vi "FPGA_w8randLEDs.vi"() -> ()   [LabVIEW 2012]
uses:
  <vilib>/Platform/TimedLoop/XDataNode/timing_clust.ctl
  <vilib>/Platform/TimedLoop/XDataNode/nitl_modes.ctl
  <vilib>/Platform/TimedLoop/XDataNode/wakeup.ctl
  <vilib>/rvi/DataTransferAndStorage/Container/Common/niFpgaContainerMetaDataKey.ctl
  <vilib>/rvi/DataTransferAndStorage/Container/Common/niFpgaContainerState.ctl
  <vilib>/rvi/DataTransferAndStorage/Container/Common/niFpgaDataTypeControl.ctl
  <vilib>/rvi/DataTransferAndStorage/Container/Common/niFpgaContainerImplementationControl.ctl
  <vilib>/rvi/DataTransferAndStorage/Container/Common/niFpgaContainerArbitrationOptionsControl.ctl
  <vilib>/rvi/DataTransferAndStorage/Container/Common/niFpgaTransferTypeControl.ctl
  <vilib>/rvi/DataTransferAndStorage/Container/Common/niFpgaContainerInitializationParameters.ctl
  <vilib>/rvi/Memory/Memory_Types/niFpgaMemoryInterfaceConfiguration.ctl
  <vilib>/rvi/FIFO/Fifo_Types/niFpgaFifoControlLogicControl.ctl
  <vilib>/rvi/eio/common/nirviEmuTemplateMethod_errors.vi
  <vilib>/rvi/FIFO/Fifo_Resource/nirvififoEmulationSetSize.vi
  <vilib>/rvi/DataTransferAndStorage/Container/Common/niFpgaContainerGetUniqueNameForEmu.vi
  <vilib>/rvi/Emulation/niFpgaSctlEmulationRegisterWithScheduler.vi
  <vilib>/rvi/Emulation/niFpgaSctlEmulationFifoFullMgr.vi
  <vilib>/rvi/errors/niFpgaSetErrorForExecOnDevCompSimple.vi
  <vilib>/rvi/eio/common/nirviEmuReportErrorAndStop.vi
  <vilib>/rvi/Memory/Memory_Emulation/nirvimemoryEmulationManagerCache_GetValue.vi
  <vilib>/rvi/Memory/Memory_Emulation/niFpgaMemoryEmulationValidateCache.vi
  <vilib>/rvi/Memory/Memory_Emulation/nirvimemoryEmulationManagerCache_InsertValue.vi
  <vilib>/rvi/Memory/Memory_Emulation/nirvimemoryEmulationManagerCache_SetValue.vi
  <vilib>/rvi/Emulation/niFpgaSctlEmulationResourceMgr.vi
  <vilib>/rvi/Memory/Memory_Emulation/niFpgaMemoryEmulationCacheClearOnFirstRun.vi
  <vilib>/rvi/Memory/Memory_Emulation/nirvimemoryEmulationManagerCache_MakeExclusive.vi
  <vilib>/rvi/Memory/Memory_Emulation/nirvimemoryEmulationManagerCache_ReleaseExclusive.vi
  <vilib>/Utility/error.llb/Clear Errors.vi
  <vilib>/rvi/Emulation/niFpgaSctlEmulationScheduler.vi
  <vilib>/rvi/DataTransferAndStorage/Container/Common/niFpgaContainerSetEmuInfo.vi
  <vilib>/eio/EIONode/EIONode.xnode
  <vilib>/rvi/DataTransferAndStorage/Container/XNode/niFpgaContainer.xnode
  <vilib>/rvi/FIFO/Fifo_Resource/nirvififoEmulationClear.vi
  <vilib>/Platform/TimedLoop/XDataNode/XDataNode.xnode
  <vilib>/rvi/FIFO/Fifo_Resource/nirvififoEmulationRead.vi
  <vilib>/rvi/DataTransferAndStorage/Register/Emulation/niFpgaRegisterEmulation.vi
  <vilib>/rvi/Memory/Memory_Emulation/nirvimemoryEmulation.vi
  <vilib>/rvi/FIFO/Fifo_Resource/nirvififoEmulationWrite.vi
  <vilib>/rvi/LocalResourceManager/LocalResourceManager.xnode
  <vilib>/Platform/TimedLoop/XDataNode/XDNodeRunTimeDep.lvlib
panel:
  out "IO Module\\ADC Error A":bool
  out "IO Module\\ADC Error B":bool
  out "IO Module\\Pll Unlocked":bool
  in  "Stop FPGA and exit":bool
  in  "Record Size only data":u32=95
  out "DMA FIFO Timed Out?":bool
  in  "circular buffer length":u32=1000
  in  "Location":i16(ring) items=["Purdue", "NIKHEF", "Zurich", "???"]
  in  "Trigger 0":i16=4000
  in  "Trigger 1":i16=4000
  in  "Trigger 2":i16=4000
  in  "Trigger 3":i16=4000
  in  "Trigger 4":i16=4000
  in  "Trigger 5":i16=4000
  in  "Trigger 6":i16=4000
  in  "Trigger 7":i16=4000
  in  "# of pretrigger":u32=20
  out "Timestamp":u64
  in  "channel 0 on/off":bool
  in  "channel 2 on/off":bool
  in  "channel 1 on/off":bool
  in  "channel 3 on/off":bool
  in  "channel 4 on/off":bool
  in  "channel 5 on/off":bool
  in  "channel 6 on/off":bool
  in  "channel 7 on/off":bool
  in  "initial value":u64
  in  "Testpulser On/Off":bool
  in  "Testpulse Time Delay (20 ns ticks)":u32=15
  in  "Testpulse duration (20 ns ticks)":u32
  out "Init Done":bool
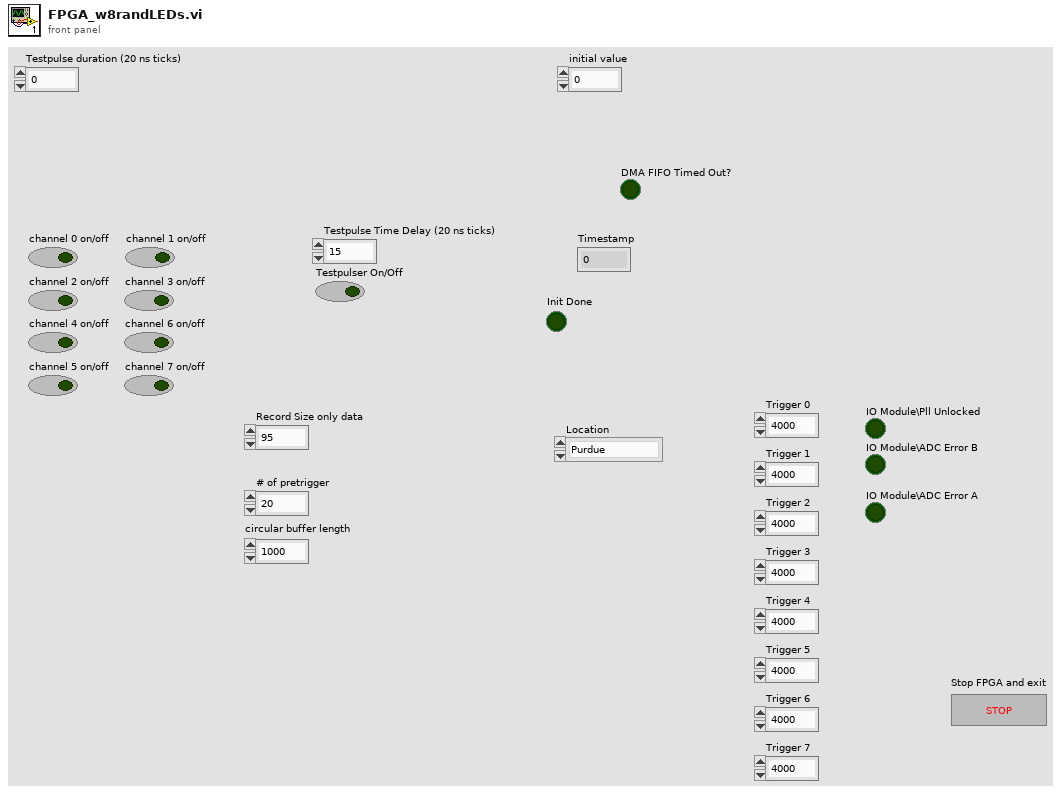
[diagram p1: front panel]
types:
  T1 = typedef "XDNodeRunTimeDep.lvlib/timing_clust.ctl" = cluster{"Expected End [f-1]":u64, "Actual End [f-1]":u64, "Finished Late? [f-1]":bool, "Expected End [i-1]":u64, "Actual End [i-1]":u64, "Finished Late? [i-1]":bool, "Expected Start [i]":u64, "Actual Start [i]":u64, "Expected Start [f]":u64, "Actual Start [f]":u64, "Source Name":string, "Structure Name":string, "Period":i64, "Deadline":i64, "Offset":i64, "Start":i64, "Priority":i32, "Timeout":i32, "Mode":T2, "Wakeup Reason":T3, "Error":errorcluster, "Source Type":string, "Secondary Source Type":string, "Global End Time":u64, "Global Start Time":u64, "Frame Duration":u64, "Iteration Duration":u64, "Assigned CPU":i32, "I/O Scan Engine Mode":u32}
  T2 = typedef "XDNodeRunTimeDep.lvlib/nitl_modes.ctl" = enum32{"No Change", "Process missed periods, maintain original phase", "Discard missed periods, maintain original phase", "Process missed periods, ignore original phase", "Discard missed periods, ignore original phase"}
  T3 = typedef "XDNodeRunTimeDep.lvlib/wakeup.ctl" = enum32{"Normal", "Aborted", "Asynchronous wakeup", "Timing source error", "Timed loop error", "Timeout"}
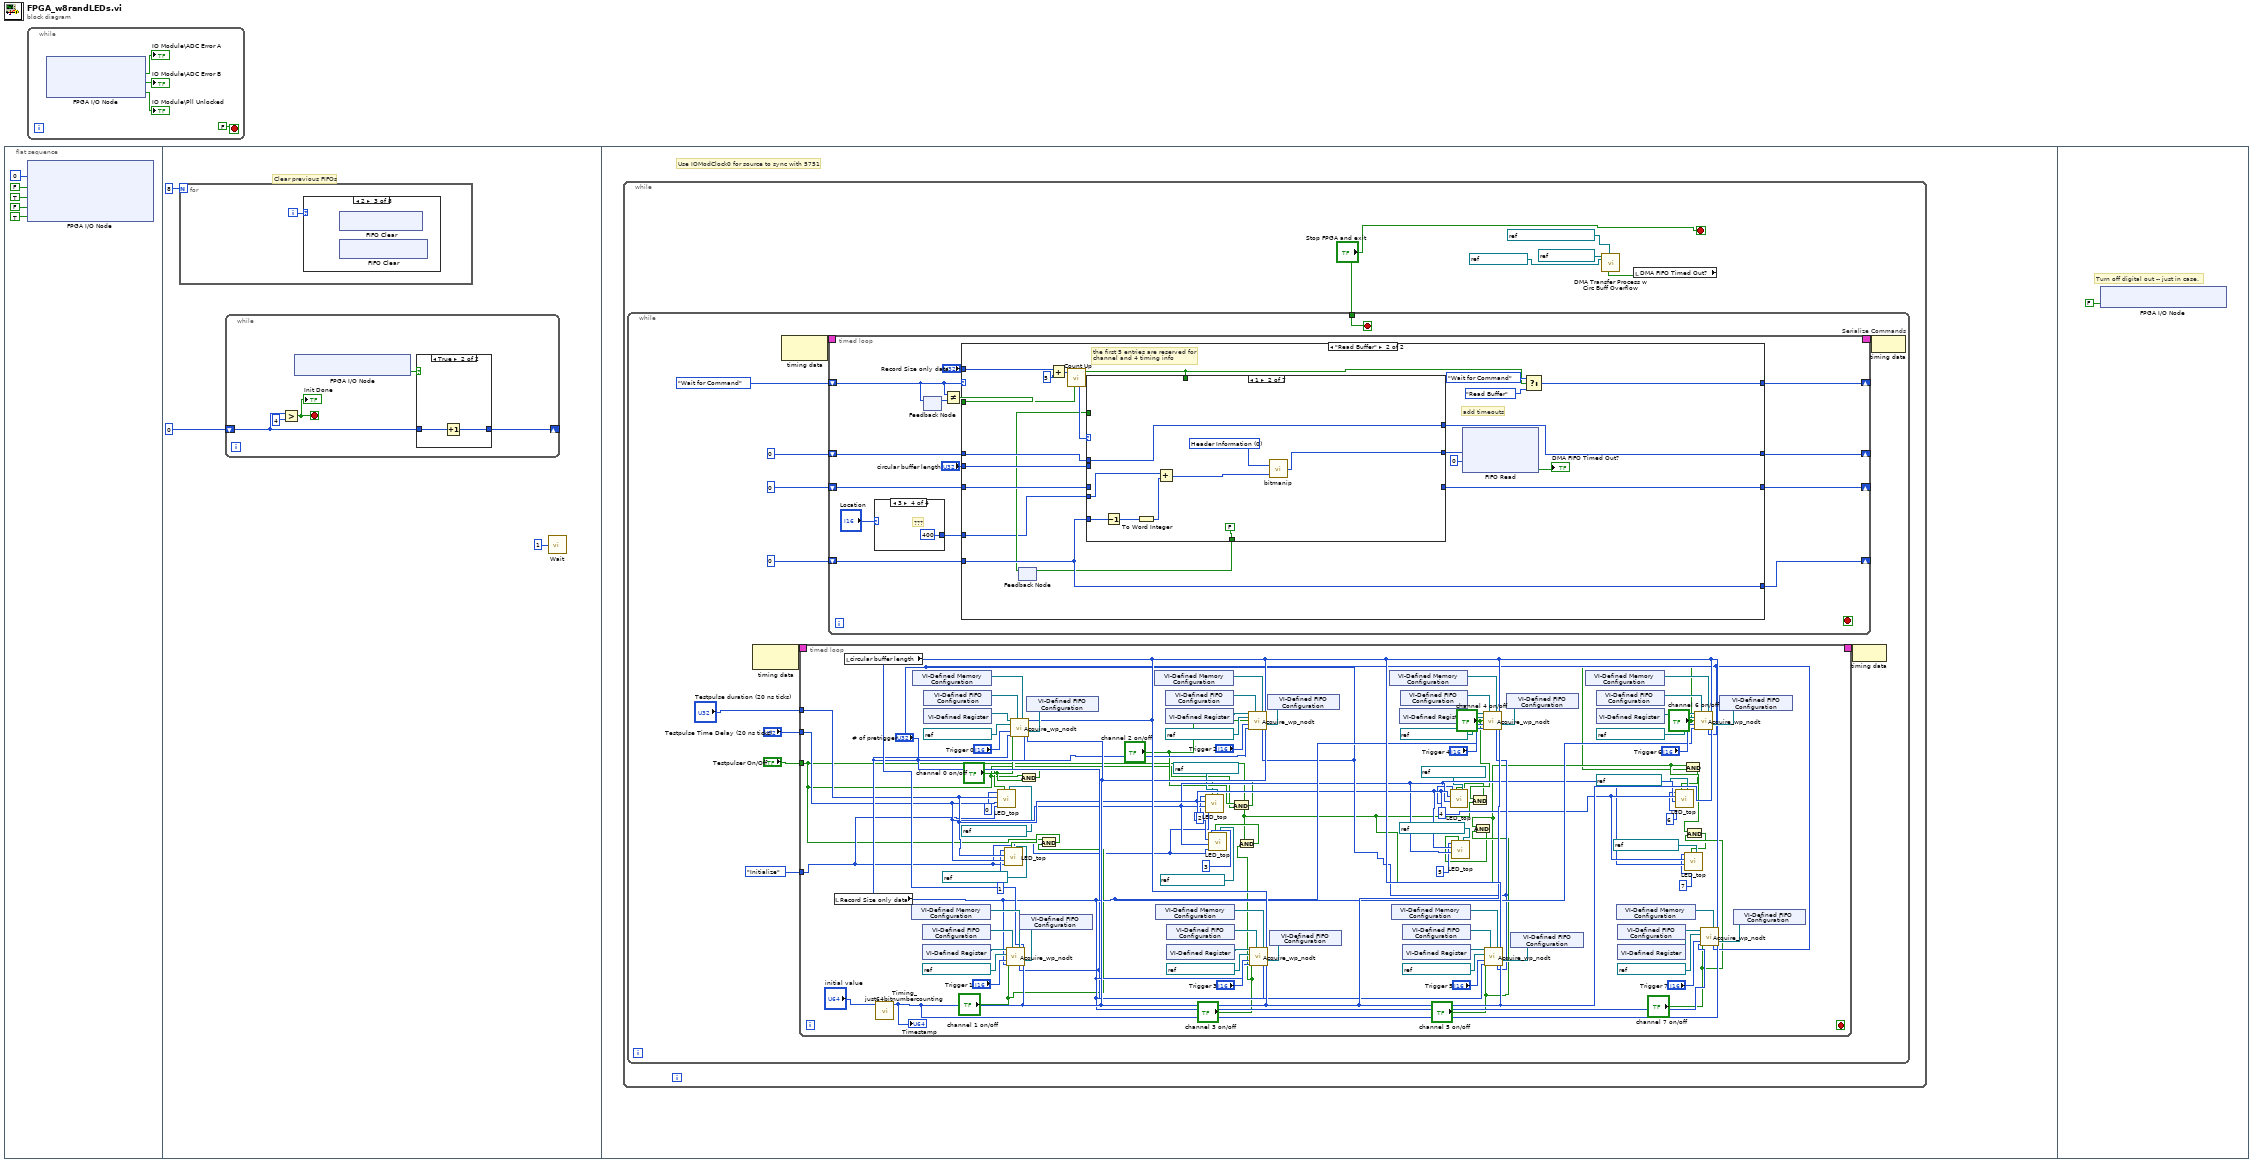
[diagram p0: block diagram]
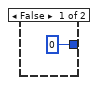
[diagram p2: hidden frame]
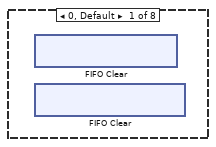
[diagram p3: hidden frame]
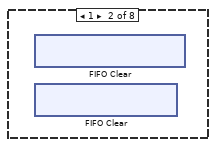
[diagram p4: hidden frame]
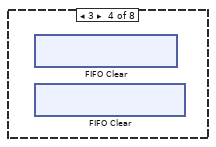
[diagram p5: hidden frame]
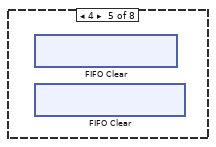
[diagram p6: hidden frame]
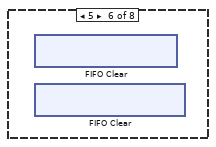
[diagram p7: hidden frame]
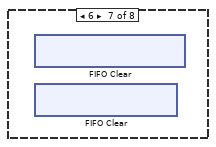
[diagram p8: hidden frame]
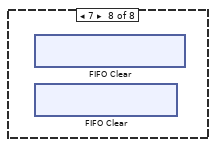
[diagram p9: hidden frame]
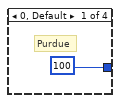
[diagram p10: hidden frame]
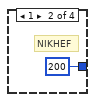
[diagram p11: hidden frame]
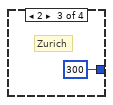
[diagram p12: hidden frame]
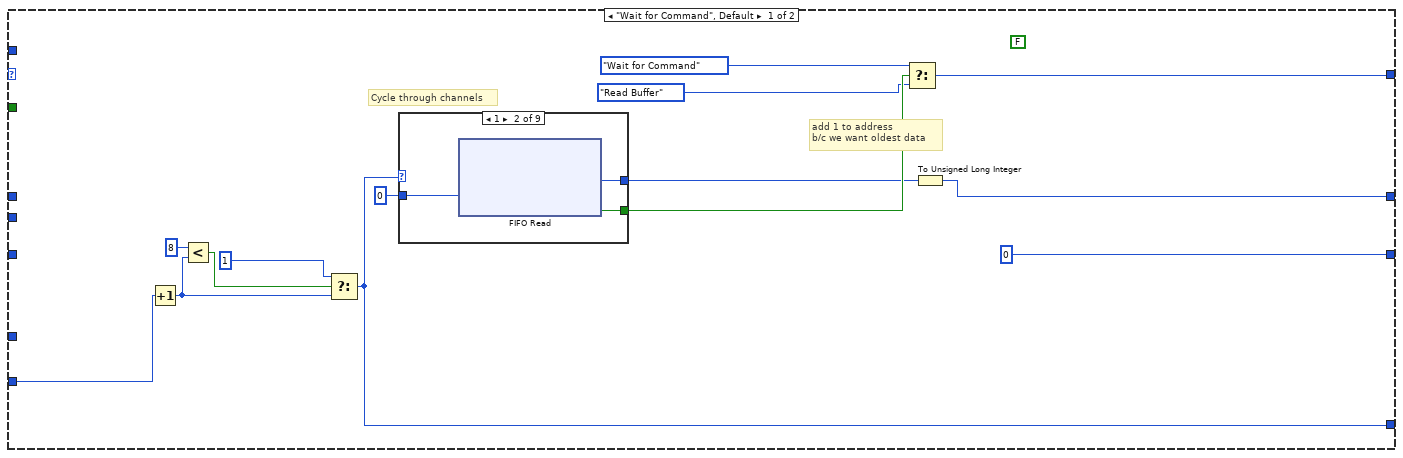
[diagram p13: hidden frame]
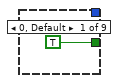
[diagram p14: hidden frame]
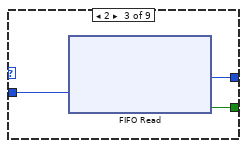
[diagram p15: hidden frame]
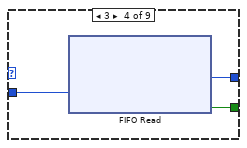
[diagram p16: hidden frame]
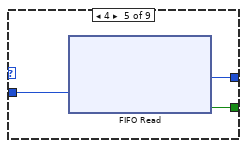
[diagram p17: hidden frame]
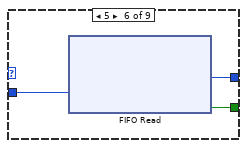
[diagram p18: hidden frame]
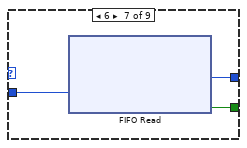
[diagram p19: hidden frame]
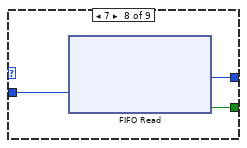
[diagram p20: hidden frame]
diagram:
  n1 = flat-sequence {
    frame #0 {
      n2 = xnode "FPGA I/O Node"("IO Module\\Sample Clock Select"=u8 0 ("IO Module\\Sample Clock Select"), "IO Module\\Force Initialization"=FALSE ("IO Module\\Force Initialization"), "IO Module\\Force Initialization"=TRUE ("IO Module\\Force Initialization"), "IO Module\\Force Initialization"=FALSE ("IO Module\\Force Initialization"), "IO Module\\Digital Output Enable"=TRUE ("IO Module\\Digital Output Enable")) -> ()  [unwired: 5 in, 5 out]
    }
    frame #1 {
      # "Clear previous FIFOs"
      n3 = for {
        N: 8 -> [_]
        i -> [w17]
        n4 = case shown="2" w17 {
          frame 0, Default {
            n5 = xnode ("FIFO Clear")() -> ()  [unwired: 1 in, 1 out]
            n6 = xnode ("FIFO Clear")() -> ()  [unwired: 1 in, 1 out]
          }
          frame 1 {
            n7 = xnode ("FIFO Clear")() -> ()  [unwired: 1 in, 1 out]
            n8 = xnode ("FIFO Clear")() -> ()  [unwired: 1 in, 1 out]
          }
          frame 2 {
            n9 = xnode ("FIFO Clear")() -> ()  [unwired: 1 in, 1 out]
            n10 = xnode ("FIFO Clear")() -> ()  [unwired: 1 in, 1 out]
          }
          frame 3 {
            n11 = xnode ("FIFO Clear")() -> ()  [unwired: 1 in, 1 out]
            n12 = xnode ("FIFO Clear")() -> ()  [unwired: 1 in, 1 out]
          }
          frame 4 {
            n13 = xnode ("FIFO Clear")() -> ()  [unwired: 1 in, 1 out]
            n14 = xnode ("FIFO Clear")() -> ()  [unwired: 1 in, 1 out]
          }
          frame 5 {
            n15 = xnode ("FIFO Clear")() -> ()  [unwired: 1 in, 1 out]
            n16 = xnode ("FIFO Clear")() -> ()  [unwired: 1 in, 1 out]
          }
          frame 6 {
            n17 = xnode ("FIFO Clear")() -> ()  [unwired: 1 in, 1 out]
            n18 = xnode ("FIFO Clear")() -> ()  [unwired: 1 in, 1 out]
          }
          frame 7 {
            n19 = xnode ("FIFO Clear")() -> ()  [unwired: 1 in, 1 out]
            n20 = xnode ("FIFO Clear")() -> ()  [unwired: 1 in, 1 out]
          }
        }
      }
      n21 = while {
        shift-right: [w12] -> _
        shift-left: u16 0 -> [w11]
        stop <- w9 stop-if-true
        n22 = Greater?(x=w11, y=u16 4) -> (0:w9:bool)
        "Init Done" <- w9
        n23 = xnode "FPGA I/O Node"() -> ("IO Module\\Initialization Done"=w13:bool)  [unwired: 1 in, 1 out]
        n24 = case shown="True" w13 {
          tunnel: [u16 0 w16] -> w12
          tunnel: w11 -> [_ w15]
          frame False {
          }
          frame True {
            n25 = Increment(x=w15) -> (x+1=w16:u16)
          }
        }
      }
      n26 = call "Wait"("Count(mSec)"=u32 1) -> ()  [unwired: 1 out]
    }
    frame #2 {
      # "Use IOModClock0 for source to sync with 5751"
      n27 = while {
        stop <- "Stop FPGA and exit" stop-if-true
        n28 = while {
          tunnel: "Stop FPGA and exit" -> [w27]
          stop <- w27 stop-if-true
          n29 = node-c288() -> (w33:T1)  [unwired: 1 in]
          n30 = node-c288() -> (w35:T1)  [unwired: 1 in]
          n31 = timed-loop {
            timing: w33 -> [_]
            timing-out: [_] -> w32
            tunnel: "Testpulser On/Off" -> [w43]
            tunnel: "Testpulse Time Delay (20 ns ticks)" -> [w71]
            tunnel: "Testpulse duration (20 ns ticks)" -> [w72]
            tunnel: enum16{"Initialize", "Get New Value", "Wait"}."Initialize" ("State In") -> [w46]
            stop <- _ stop-if-true
            n32 = local read "Record Size only data"() -> (w75:u32)
            n33 = local read "circular buffer length"() -> (w77:u32)
            n34 = call "Timing_just64bitnumbercounting.vi"("initial value"="initial value") -> ("x+1"=w76:u64)  [unwired: 10 in]
            "Timestamp" <- w76
            n35 = xnode "VI-Defined Memory Configuration"() -> ("Memory Out"=w123:refnum<k21>)
            n36 = xnode "VI-Defined Memory Configuration"() -> ("Memory Out"=w78:refnum<k21>)
            n37 = xnode "VI-Defined FIFO Configuration"() -> ("FIFO Out"=w122:refnum<k21>)
            n38 = xnode "VI-Defined Register"() -> ("Register Out"=w103:refnum<k21>)
            n39 = xnode "VI-Defined FIFO Configuration"() -> ("FIFO Out"=w79:refnum<k21>)
            n40 = xnode "VI-Defined Register"() -> ("Register Out"=w74:refnum<k21>)
            n41 = xnode "VI-Defined FIFO Configuration"() -> ("FIFO Out"=w89:refnum<k21>)
            n42 = call "Acquire_wp_nodt.vi"("Ch Armed Reg"=w103, "Command FIFO"=w122, "Circular Buffer Mem"=w123, "circular buffer length"=w77, "FPGA I/O In"=refnum<k21> "IO Module\\AI A1", "channel on/off"="channel 1 on/off", "Trigger"="Trigger 1", "Timing FIFO"=w89, "Samples to Acquire"=w75, "# of pretrigger"="# of pretrigger", "timing"=w76) -> ()  [unwired: 5 in]
            n43 = And(x=w43, y="channel 0 on/off") -> (x .and. y?=w54:bool)
            n44 = call "LED_top.vi"("FPGA I/O In"=refnum<k21> "IO Module\\D0 0", "Testpulser On/Off"=w54, "State In"=w46, "Testpulse Time Delay (20 ns ticks)"=w71, "Testpulse duration (20 ns ticks)"=w72, "Address In"=u16 0 ("Total number of pulses sent")) -> ()  [unwired: 4 in, 2 out]
            n45 = xnode "VI-Defined FIFO Configuration"() -> ("FIFO Out"=w82:refnum<k21>)
            n46 = call "Acquire_wp_nodt.vi"("Ch Armed Reg"=w74, "Command FIFO"=w79, "Circular Buffer Mem"=w78, "circular buffer length"=w77, "FPGA I/O In"=refnum<k21> "IO Module\\AI A0", "channel on/off"="channel 0 on/off", "Trigger"="Trigger 0", "Timing FIFO"=w82, "Samples to Acquire"=w75, "# of pretrigger"="# of pretrigger", "timing"=w76) -> ()  [unwired: 5 in]
            n47 = And(x=w43, y="channel 1 on/off") -> (x .and. y?=w52:bool)
            n48 = call "LED_top.vi"("FPGA I/O In"=refnum<k21> "IO Module\\D0 1", "Testpulser On/Off"=w52, "State In"=w46, "Testpulse Time Delay (20 ns ticks)"=w71, "Testpulse duration (20 ns ticks)"=w72, "Address In"=u16 1) -> ()  [unwired: 4 in, 2 out]
            n49 = xnode "VI-Defined Memory Configuration"() -> ("Memory Out"=w117:refnum<k21>)
            n50 = xnode "VI-Defined Memory Configuration"() -> ("Memory Out"=w120:refnum<k21>)
            n51 = xnode "VI-Defined FIFO Configuration"() -> ("FIFO Out"=w116:refnum<k21>)
            n52 = xnode "VI-Defined Register"() -> ("Register Out"=w99:refnum<k21>)
            n53 = xnode "VI-Defined FIFO Configuration"() -> ("FIFO Out"=w121:refnum<k21>)
            n54 = xnode "VI-Defined Register"() -> ("Register Out"=w101:refnum<k21>)
            n55 = And(x="channel 2 on/off", y=w43) -> (x .and. y?=w50:bool)
            n56 = call "LED_top.vi"("FPGA I/O In"=refnum<k21> "IO Module\\D0 2", "Testpulser On/Off"=w50, "State In"=w46, "Testpulse Time Delay (20 ns ticks)"=w71, "Testpulse duration (20 ns ticks)"=w72, "Address In"=u16 2 ("Total number of pulses sent")) -> ()  [unwired: 4 in, 2 out]
            n57 = And(x=w43, y="channel 3 on/off") -> (x .and. y?=w47:bool)
            n58 = call "LED_top.vi"("FPGA I/O In"=refnum<k21> "IO Module\\D0 3", "Testpulser On/Off"=w47, "State In"=w46, "Testpulse Time Delay (20 ns ticks)"=w71, "Testpulse duration (20 ns ticks)"=w72, "Address In"=u16 3 ("Total number of pulses sent")) -> ()  [unwired: 4 in, 2 out]
            n59 = xnode "VI-Defined FIFO Configuration"() -> ("FIFO Out"=w88:refnum<k21>)
            n60 = call "Acquire_wp_nodt.vi"("Ch Armed Reg"=w99, "Command FIFO"=w116, "Circular Buffer Mem"=w117, "circular buffer length"=w77, "FPGA I/O In"=refnum<k21> "IO Module\\AI A2", "channel on/off"="channel 2 on/off", "Trigger"="Trigger 2", "Timing FIFO"=w88, "Samples to Acquire"=w75, "# of pretrigger"="# of pretrigger", "timing"=w76) -> ()  [unwired: 5 in]
            n61 = xnode "VI-Defined FIFO Configuration"() -> ("FIFO Out"=w87:refnum<k21>)
            n62 = call "Acquire_wp_nodt.vi"("Ch Armed Reg"=w101, "Command FIFO"=w121, "Circular Buffer Mem"=w120, "circular buffer length"=w77, "FPGA I/O In"=refnum<k21> "IO Module\\AI A3", "channel on/off"="channel 3 on/off", "Trigger"="Trigger 3", "Timing FIFO"=w87, "Samples to Acquire"=w75, "# of pretrigger"="# of pretrigger", "timing"=w76) -> ()  [unwired: 5 in]
            n63 = xnode "VI-Defined Memory Configuration"() -> ("Memory Out"=w105:refnum<k21>)
            n64 = xnode "VI-Defined Memory Configuration"() -> ("Memory Out"=w108:refnum<k21>)
            n65 = xnode "VI-Defined Register"() -> ("Register Out"=w93:refnum<k21>)
            n66 = xnode "VI-Defined FIFO Configuration"() -> ("FIFO Out"=w104:refnum<k21>)
            n67 = xnode "VI-Defined FIFO Configuration"() -> ("FIFO Out"=w109:refnum<k21>)
            n68 = xnode "VI-Defined Register"() -> ("Register Out"=w97:refnum<k21>)
            n69 = And(x="channel 4 on/off", y=w43) -> (x .and. y?=w42:bool)
            n70 = call "LED_top.vi"("FPGA I/O In"=refnum<k21> "IO Module\\D0 4", "Testpulser On/Off"=w42, "Testpulse Time Delay (20 ns ticks)"=w71, "Testpulse duration (20 ns ticks)"=w72, "Address In"=u16 4 ("Total number of pulses sent")) -> ()  [unwired: 5 in, 2 out]
            n71 = And(x=w43, y="channel 5 on/off") -> (x .and. y?=w41:bool)
            n72 = call "LED_top.vi"("FPGA I/O In"=refnum<k21> "IO Module\\D0 5", "Testpulser On/Off"=w41, "Testpulse Time Delay (20 ns ticks)"=w71, "Testpulse duration (20 ns ticks)"=w72, "Address In"=u16 5 ("Total number of pulses sent")) -> ()  [unwired: 5 in, 2 out]
            n73 = xnode "VI-Defined FIFO Configuration"() -> ("FIFO Out"=w86:refnum<k21>)
            n74 = call "Acquire_wp_nodt.vi"("Ch Armed Reg"=w93, "Command FIFO"=w104, "Circular Buffer Mem"=w105, "circular buffer length"=w77, "FPGA I/O In"=refnum<k21> "IO Module\\AI A4", "channel on/off"="channel 4 on/off", "Trigger"="Trigger 4", "Timing FIFO"=w86, "Samples to Acquire"=w75, "# of pretrigger"="# of pretrigger", "timing"=w76) -> ()  [unwired: 5 in]
            n75 = xnode "VI-Defined FIFO Configuration"() -> ("FIFO Out"=w85:refnum<k21>)
            n76 = call "Acquire_wp_nodt.vi"("Ch Armed Reg"=w97, "Command FIFO"=w109, "Circular Buffer Mem"=w108, "circular buffer length"=w77, "FPGA I/O In"=refnum<k21> "IO Module\\AI A5", "channel on/off"="channel 5 on/off", "Trigger"="Trigger 5", "Timing FIFO"=w85, "Samples to Acquire"=w75, "# of pretrigger"="# of pretrigger", "timing"=w76) -> ()  [unwired: 5 in]
            n77 = xnode "VI-Defined Memory Configuration"() -> ("Memory Out"=w114:refnum<k21>)
            n78 = xnode "VI-Defined FIFO Configuration"() -> ("FIFO Out"=w115:refnum<k21>)
            n79 = xnode "VI-Defined Register"() -> ("Register Out"=w95:refnum<k21>)
            n80 = xnode "VI-Defined Memory Configuration"() -> ("Memory Out"=w111:refnum<k21>)
            n81 = xnode "VI-Defined FIFO Configuration"() -> ("FIFO Out"=w110:refnum<k21>)
            n82 = xnode "VI-Defined Register"() -> ("Register Out"=w91:refnum<k21>)
            n83 = And(x=w43, y="channel 6 on/off") -> (x .and. y?=w37:bool)
            n84 = call "LED_top.vi"("FPGA I/O In"=refnum<k21> "IO Module\\D0 6", "Testpulser On/Off"=w37, "Testpulse Time Delay (20 ns ticks)"=w71, "Testpulse duration (20 ns ticks)"=w72, "Address In"=u16 6 ("Total number of pulses sent")) -> ()  [unwired: 5 in, 2 out]
            n85 = And(x=w43, y="channel 7 on/off") -> (x .and. y?=w38:bool)
            n86 = call "LED_top.vi"("FPGA I/O In"=refnum<k21> "IO Module\\D0 7", "Testpulser On/Off"=w38, "Testpulse Time Delay (20 ns ticks)"=w71, "Testpulse duration (20 ns ticks)"=w72, "Address In"=u16 7 ("Total number of pulses sent")) -> ()  [unwired: 5 in, 2 out]
            n87 = xnode "VI-Defined FIFO Configuration"() -> ("FIFO Out"=w84:refnum<k21>)
            n88 = call "Acquire_wp_nodt.vi"("Ch Armed Reg"=w95, "Command FIFO"=w115, "Circular Buffer Mem"=w114, "circular buffer length"=w77, "FPGA I/O In"=refnum<k21> "IO Module\\AI A6", "channel on/off"="channel 6 on/off", "Trigger"="Trigger 6", "Timing FIFO"=w84, "Samples to Acquire"=w75, "# of pretrigger"="# of pretrigger", "timing"=w76) -> ()  [unwired: 5 in]
            n89 = xnode "VI-Defined FIFO Configuration"() -> ("FIFO Out"=w83:refnum<k21>)
            n90 = call "Acquire_wp_nodt.vi"("Ch Armed Reg"=w91, "Command FIFO"=w110, "Circular Buffer Mem"=w111, "circular buffer length"=w77, "FPGA I/O In"=refnum<k21> "IO Module\\AI A7", "channel on/off"="channel 7 on/off", "Trigger"="Trigger 7", "Timing FIFO"=w83, "Samples to Acquire"=w75, "# of pretrigger"="# of pretrigger", "timing"=w76) -> ()  [unwired: 5 in]
          }
          n91 = timed-loop "Serialize Commands" {
            timing: w35 -> [_]
            timing-out: [_] -> w34
            shift-right: [w905] -> _
            shift-left: enum16{"Wait for Command", "Read Buffer"}."Wait for Command" -> [w903]
            shift-right: [w909] -> _
            shift-left: u32 0 ("Element") -> [w908]
            shift-right: [w907] -> _
            shift-left: u8 0 ("t") -> [w906]
            shift-right: [w900] -> _
            shift-left: u64 0 ("Element") -> [w899]
            stop <- _ stop-if-true
            n92 = case shown="3" "Location" {
              tunnel: [i16 100 i16 200 i16 300 i16 400] -> w898
              frame 0, Default {
                # "Purdue"
              }
              frame 1 {
                # "NIKHEF"
              }
              frame 2 {
                # "Zurich"
              }
              frame 3 {
                # "???"
              }
            }
            n93 = feedback-in #1(w903) -> ()
            n94 = feedback #1() -> (w904:enum16{"Wait for Command", "Read Buffer"})  [unwired: 1 in]
            n95 = Not Equal?(x=w903, y=w904) -> (x != y?=w901:bool)
            n96 = case shown="\"Read Buffer\"" w903 {
              tunnel: "Record Size only data" -> [_ w963]
              tunnel: [w917 w973] -> w907
              tunnel: w906 -> [w919 w973]
              tunnel: [w920 w958] -> w909
              tunnel: w908 -> [_ w972]
              tunnel: [w923 w974] -> w905
              tunnel: "circular buffer length" -> [_ w971]
              tunnel: w901 -> [_ w965]
              tunnel: [u64 0 ("Element") w960] -> w900
              tunnel: w899 -> [_ w959]
              tunnel: w898 -> [_ w954]
              frame "Wait for Command", Default {
                (unwired) FALSE
                # "add 1 to address\nb/c we want oldest data"
                # "Cycle through channels"
                n97 = Increment(x=w919) -> (x+1=w918:u8)
                n98 = Less?(x=u8 8, y=w918) -> (x < y?=w927:bool)
                n99 = Select(t=u8 1, s=w927, f=w918) -> (s? t:f=w917:u8)
                n100 = case shown="1" w917 {
                  tunnel: [TRUE ("Timed Out?") w932 w933 w936 w939 w942 w945 w948 w951] -> w924
                  tunnel: 0 ("Timeout") -> [_ w931 w935 w938 w941 w944 w947 w950 w953]
                  tunnel: [_ w930 w934 w937 w940 w943 w946 w949 w952] -> w916
                  frame 0, Default {
                  }
                  frame 1 {
                    n101 = xnode ("FIFO Read")("Timeout"=w931) -> ("Element"=w930:i16, "Timed Out?"=w932:bool)  [unwired: 1 in, 1 out]
                  }
                  frame 2 {
                    n102 = xnode ("FIFO Read")("Timeout"=w935) -> ("Element"=w934:i16, "Timed Out?"=w933:bool)  [unwired: 1 in, 1 out]
                  }
                  frame 3 {
                    n103 = xnode ("FIFO Read")("Timeout"=w938) -> ("Element"=w937:i16, "Timed Out?"=w936:bool)  [unwired: 1 in, 1 out]
                  }
                  frame 4 {
                    n104 = xnode ("FIFO Read")("Timeout"=w941) -> ("Element"=w940:i16, "Timed Out?"=w939:bool)  [unwired: 1 in, 1 out]
                  }
                  frame 5 {
                    n105 = xnode ("FIFO Read")("Timeout"=w944) -> ("Element"=w943:i16, "Timed Out?"=w942:bool)  [unwired: 1 in, 1 out]
                  }
                  frame 6 {
                    n106 = xnode ("FIFO Read")("Timeout"=w947) -> ("Element"=w946:i16, "Timed Out?"=w945:bool)  [unwired: 1 in, 1 out]
                  }
                  frame 7 {
                    n107 = xnode ("FIFO Read")("Timeout"=w950) -> ("Element"=w949:i16, "Timed Out?"=w948:bool)  [unwired: 1 in, 1 out]
                  }
                  frame 8 {
                    n108 = xnode ("FIFO Read")("Timeout"=w953) -> ("Element"=w952:i16, "Timed Out?"=w951:bool)  [unwired: 1 in, 1 out]
                  }
                }
                n109 = Select(t=enum16{"Wait for Command", "Read Buffer"}."Wait for Command", s=w924, f=enum16{"Wait for Command", "Read Buffer"}."Read Buffer") -> (s? t:f=w923:enum16{"Wait for Command", "Read Buffer"})
                n110 = To Unsigned Long Integer(number=w916) -> (unsigned 32bit integer=w920:u32)
              }
              frame "Read Buffer" {
                # "the first 5 entries are reserved for channel and 4 timing info"
                # "add timeouts"
                n111 = feedback #2() -> (w957:bool)  [unwired: 1 in]
                n112 = Add(x=w963, y=u32 5) -> (x+y=w961:u32)
                n113 = call "Count Up.vi"("Reset?"=w965, "goal"=w961) -> ("Count Met"=w967:bool, "count"=w964:u32)  [unwired: 8 in]
                n114 = case shown="1" w964 {
                  tunnel: w973 -> [_ w981 w990 _ _ _ w1029]
                  tunnel: w972 -> [_ w987 w992 w1013 w1019 w1025 w1036]
                  tunnel: w971 -> [_ _ _ _ _ _ w1035]
                  tunnel: w967 -> [_ _ _ _ _ _ w1034]
                  tunnel: [i16 0 ("Data") w984 w994 w1011 w1017 w1023 w1030] -> w966
                  tunnel: w957 -> [_ _ _ _ _ _ w1032]
                  tunnel: [u64 0 ("Element") _ w991 w1014 w1020 w1026 _] -> w960
                  tunnel: w959 -> [_ _ _ w1014 w1020 w1026 _]
                  tunnel: [u32 0 ("Element") w987 w992 w1013 w1019 w1025 _] -> w958
                  tunnel: [FALSE FALSE FALSE FALSE FALSE TRUE FALSE] -> w956
                  tunnel: w954 -> [_ w979 _ _ _ _ _]
                  frame 0, Default {
                  }
                  frame 1 {
                    w983 = u16 0 items=["Header Information", "Particle Pulse", "Test Pulse"] ("Pulse Type")
                    n115 = Decrement(x=w981) -> (x-1=w982:u8)
                    n116 = To Word Integer(number=w982) -> (16bit integer=w980:i16)
                    n117 = Add(x=w979, y=w980) -> (x+y=w985:i16)
                    n118 = call "bitmanip.vi"("Pulse Type"=w983, "Integer to be written"=w985) -> ("Integer Written"=w984:i16)  [unwired: 2 in]
                  }
                  frame 2 {
                    # "reads out the lsb of the timing information"
                    n119 = case shown="2" w990 {
                      tunnel: [_ w995 w997 w999 w1001 w1003 w1005 w1007 w1009] -> w991
                      frame Default {
                      }
                      frame 1 {
                        n120 = xnode ("FIFO Read")("Timeout"=0) -> ("Element"=w995:u64)  [unwired: 1 in, 2 out]
                      }
                      frame 2 {
                        n121 = xnode ("FIFO Read")("Timeout"=0) -> ("Element"=w997:u64)  [unwired: 1 in, 2 out]
                      }
                      frame 3 {
                        n122 = xnode ("FIFO Read")("Timeout"=0) -> ("Element"=w999:u64)  [unwired: 1 in, 2 out]
                      }
                      frame 4 {
                        n123 = xnode ("FIFO Read")("Timeout"=0) -> ("Element"=w1001:u64)  [unwired: 1 in, 2 out]
                      }
                      frame 5 {
                        n124 = xnode ("FIFO Read")("Timeout"=0) -> ("Element"=w1003:u64)  [unwired: 1 in, 2 out]
                      }
                      frame 6 {
                        n125 = xnode ("FIFO Read")("Timeout"=0) -> ("Element"=w1005:u64)  [unwired: 1 in, 2 out]
                      }
                      frame 7 {
                        n126 = xnode ("FIFO Read")("Timeout"=0) -> ("Element"=w1007:u64)  [unwired: 1 in, 2 out]
                      }
                      frame 8 {
                        n127 = xnode ("FIFO Read")("Timeout"=0) -> ("Element"=w1009:u64)  [unwired: 1 in, 2 out]
                      }
                    }
                    n128 = Split Number(x=w991) -> (hi(x)=w989:u32)  [unwired: 1 out]
                    n129 = Split Number(x=w989) -> (hi(x)=w988:u16)  [unwired: 1 out]
                    n130 = To Word Integer(number=w988) -> (16bit integer=w994:i16)
                  }
                  frame 3 {
                    n131 = Split Number(x=w1014) -> (hi(x)=w1016:u32)  [unwired: 1 out]
                    n132 = Split Number(x=w1016) -> (lo(x)=w1015:u16)  [unwired: 1 out]
                    n133 = To Word Integer(number=w1015) -> (16bit integer=w1011:i16)
                  }
                  frame 4 {
                    n134 = Split Number(x=w1020) -> (lo(x)=w1022:u32)  [unwired: 1 out]
                    n135 = Split Number(x=w1022) -> (hi(x)=w1021:u16)  [unwired: 1 out]
                    n136 = To Word Integer(number=w1021) -> (16bit integer=w1017:i16)
                  }
                  frame 5 {
                    n137 = Split Number(x=w1026) -> (lo(x)=w1028:u32)  [unwired: 1 out]
                    n138 = Split Number(x=w1028) -> (lo(x)=w1027:u16)  [unwired: 1 out]
                    n139 = To Word Integer(number=w1027) -> (16bit integer=w1023:i16)
                  }
                  frame 6.. {
                    n140 = call "Circular Buffer Address_try_without_deadtime.vi"("Reset?"=w1032, "Starting Address"=w1036, "circular buffer length"=w1035) -> ("Address"=w1033:u32)  [unwired: 8 in]
                    n141 = case shown="1" w1029 {
                      tunnel: w1033 -> [_ w1040 w1043 w1046 w1049 w1052 w1055 w1058 w1061]
                      tunnel: w1034 -> [_ w1039 w1042 w1045 w1048 w1051 w1054 w1057 w1060]
                      tunnel: [i16 0 w1038 w1041 w1044 w1047 w1050 w1053 w1056 w1059] -> w1030
                      frame Default {
                        # "Error"
                      }
                      frame 1 {
                        n142 = xnode ("Memory Read")("Address"=w1040) -> ("Data"=w1038:i16)  [unwired: 1 in, 1 out]
                        n143 = xnode ("Register Write")("Data"=w1039) -> ()  [unwired: 1 in, 1 out]
                      }
                      frame 2 {
                        n144 = xnode ("Memory Read")("Address"=w1043) -> ("Data"=w1041:i16)  [unwired: 1 in, 1 out]
                        n145 = xnode ("Register Write")("Data"=w1042) -> ()  [unwired: 1 in, 1 out]
                      }
                      frame 3 {
                        n146 = xnode ("Memory Read")("Address"=w1046) -> ("Data"=w1044:i16)  [unwired: 1 in, 1 out]
                        n147 = xnode ("Register Write")("Data"=w1045) -> ()  [unwired: 1 in, 1 out]
                      }
                      frame 4 {
                        n148 = xnode ("Memory Read")("Address"=w1049) -> ("Data"=w1047:i16)  [unwired: 1 in, 1 out]
                        n149 = xnode ("Register Write")("Data"=w1048) -> ()  [unwired: 1 in, 1 out]
                      }
                      frame 5 {
                        n150 = xnode ("Memory Read")("Address"=w1052) -> ("Data"=w1050:i16)  [unwired: 1 in, 1 out]
                        n151 = xnode ("Register Write")("Data"=w1051) -> ()  [unwired: 1 in, 1 out]
                      }
                      frame 6 {
                        n152 = xnode ("Memory Read")("Address"=w1055) -> ("Data"=w1053:i16)  [unwired: 1 in, 1 out]
                        n153 = xnode ("Register Write")("Data"=w1054) -> ()  [unwired: 1 in, 1 out]
                      }
                      frame 7 {
                        n154 = xnode ("Memory Read")("Address"=w1058) -> ("Data"=w1056:i16)  [unwired: 1 in, 1 out]
                        n155 = xnode ("Register Write")("Data"=w1057) -> ()  [unwired: 1 in, 1 out]
                      }
                      frame 8 {
                        n156 = xnode ("Memory Read")("Address"=w1061) -> ("Data"=w1059:i16)  [unwired: 1 in, 1 out]
                        n157 = xnode ("Register Write")("Data"=w1060) -> ()  [unwired: 1 in, 1 out]
                      }
                    }
                  }
                }
                n158 = feedback-in #2(w956) -> ()
                n159 = xnode ("FIFO Read")("Element"=w966, "Timeout"=0) -> ("Timed Out?"=→"DMA FIFO Timed Out?":bool)  [unwired: 1 in, 1 out]
                n160 = Select(t=enum16{"Wait for Command", "Read Buffer"}."Wait for Command", s=w967, f=enum16{"Wait for Command", "Read Buffer"}."Read Buffer") -> (s? t:f=w974:enum16{"Wait for Command", "Read Buffer"})
              }
            }
          }
          n161 = node-c288(w32) -> ()
          n162 = node-c288(w34) -> ()
        }
        n163 = local read "DMA FIFO Timed Out?"() -> (w20:bool)
        n164 = call "DMA Transfer Process w Circ Buff Overflow.vi"("DMA Write Timed Out?"=w20, "Clock Domain"=refnum<k21> "40 MHz Onboard Clock", "Local"=refnum<k21> "To DMA FIFO", "DMA"=refnum<k21> "To Host FIFO") -> ()  [unwired: 8 in]
      }
    }
    frame #3 {
      # "Turn off digital out -- just in case."
      n165 = xnode "FPGA I/O Node"("IO Module\\Digital Output Enable"=FALSE ("IO Module\\Digital Output Enable")) -> ()  [unwired: 1 in, 1 out]
    }
  }
  n166 = while {
    stop <- FALSE stop-if-true
    n167 = xnode "FPGA I/O Node"() -> ("IO Module\\ADC Error A"=→"IO Module\\ADC Error A":bool, "IO Module\\ADC Error B"=→"IO Module\\ADC Error B":bool, "IO Module\\Pll Unlocked"=→"IO Module\\Pll Unlocked":bool)  [unwired: 3 in, 3 out]
  }
